vi "Avarage_measurements.vi"() -> ()   [LabVIEW 2015]
uses:
  <vilib>/Analysis/NI_AALBase.lvlib
panel:
  out "output cluster 2":T1
  out "output cluster":T1
  in  "Measurement Arrays 2":T1
  in  "Measurement Arrays":T2
  out "Stdev Measurements":T2
  out "Averaged Measurements":T2
  out "Change index":u16[](array[numeric])
  out "N":u16
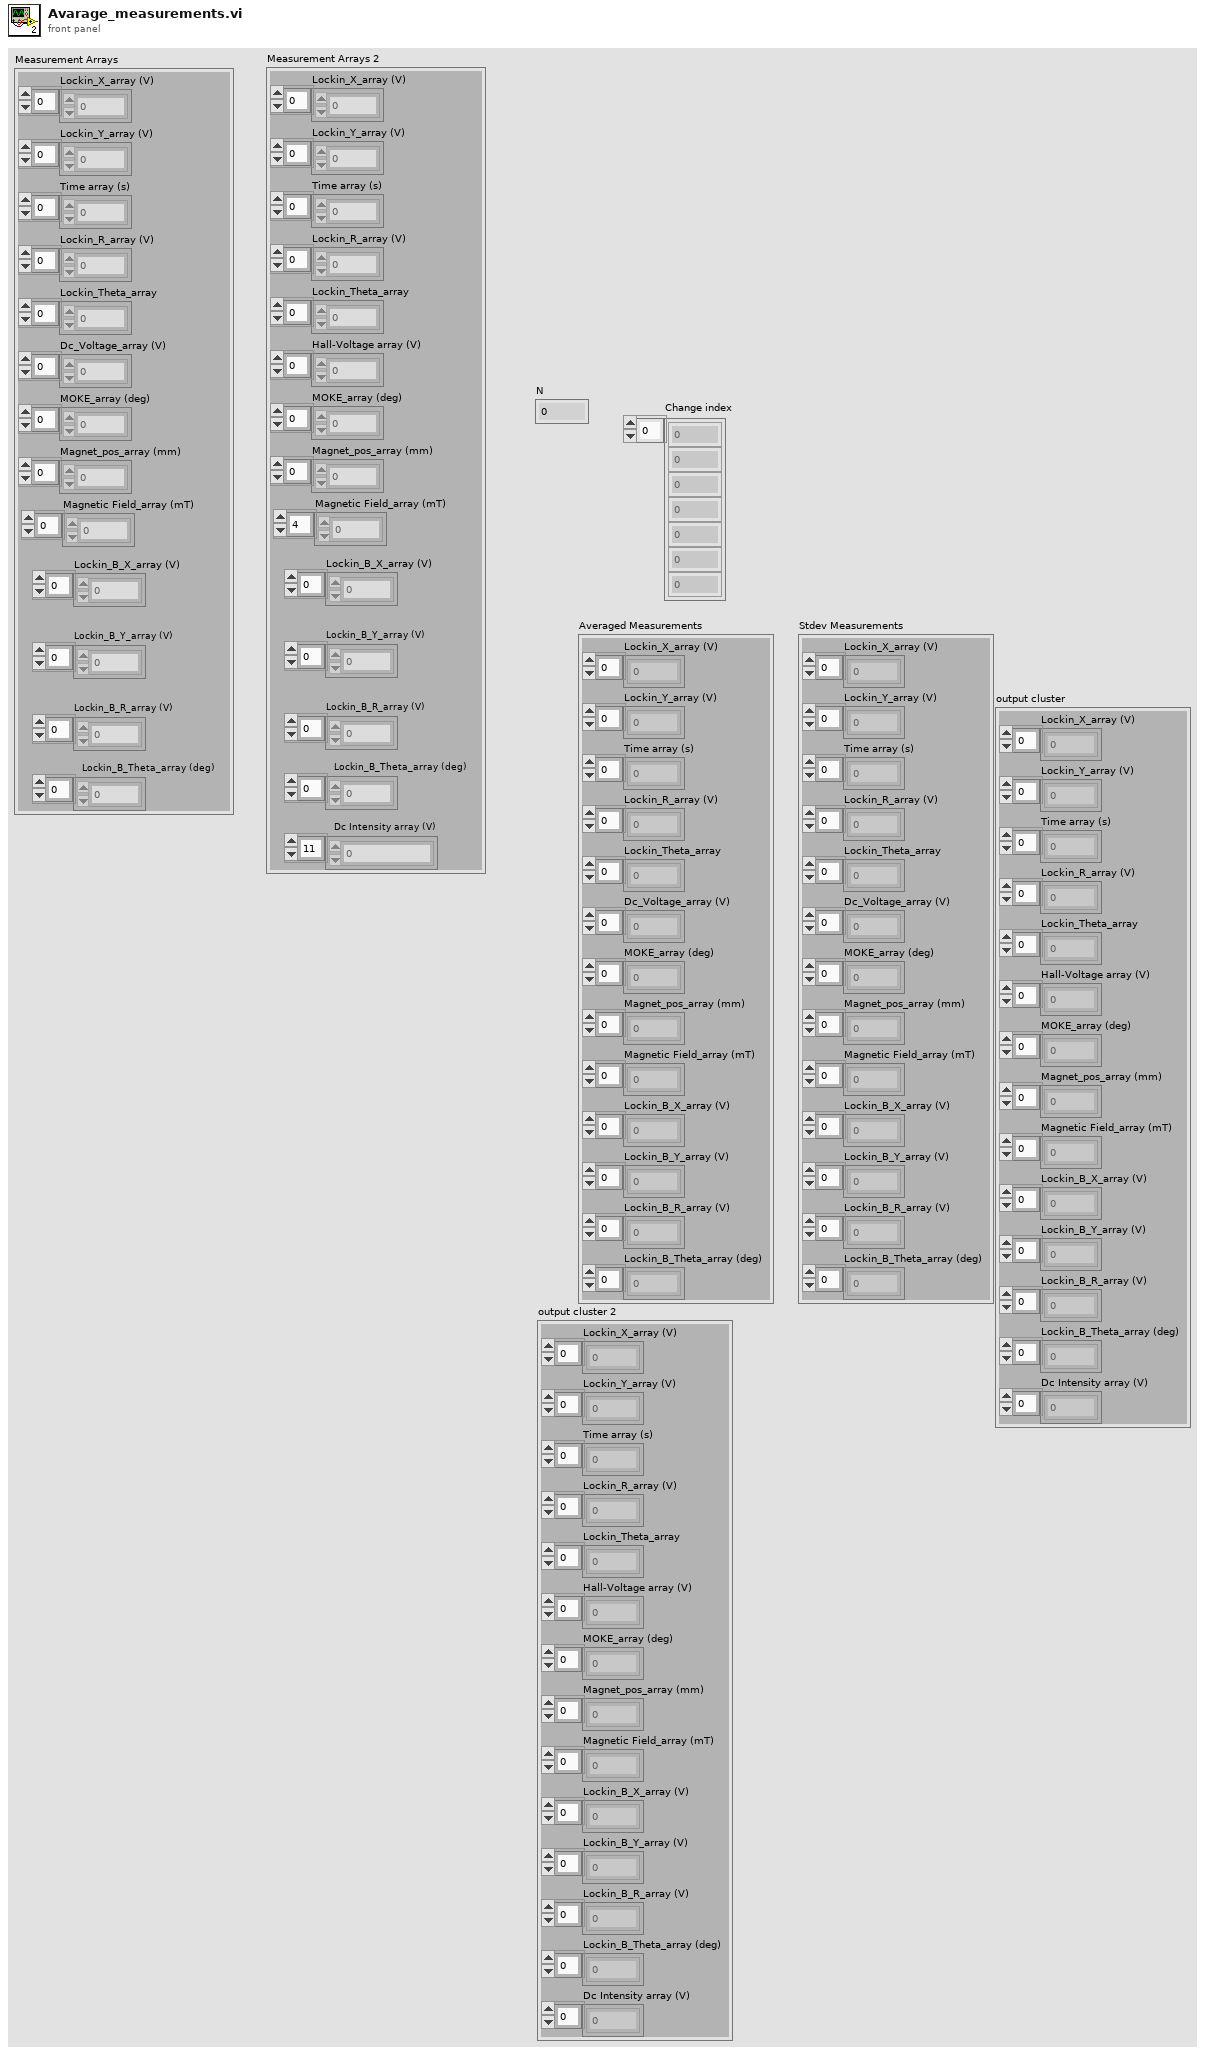
[diagram p1: front panel]
types:
  T1 = cluster{"Lockin_X_array (V)":dbl[], "Lockin_Y_array (V)":dbl[], "Time array (s)":dbl[], "Lockin_R_array (V)":dbl[], "Lockin_Theta_array":dbl[], "Hall-Voltage array (V)":dbl[], "MOKE_array (deg)":dbl[], "Magnet_pos_array (mm)":dbl[], "Magnetic Field_array (mT)":dbl[], "Lockin_B_X_array (V)":dbl[], "Lockin_B_Y_array (V)":dbl[], "Lockin_B_R_array (V)":dbl[], "Lockin_B_Theta_array (deg)":dbl[], "Dc Intensity array (V)":dbl[]}
  T2 = cluster{"Lockin_X_array (V)":dbl[], "Lockin_Y_array (V)":dbl[], "Time array (s)":dbl[], "Lockin_R_array (V)":dbl[], "Lockin_Theta_array":dbl[], "Dc_Voltage_array (V)":dbl[], "MOKE_array (deg)":dbl[], "Magnet_pos_array (mm)":dbl[], "Magnetic Field_array (mT)":dbl[], "Lockin_B_X_array (V)":dbl[], "Lockin_B_Y_array (V)":dbl[], "Lockin_B_R_array (V)":dbl[], "Lockin_B_Theta_array (deg)":dbl[]}
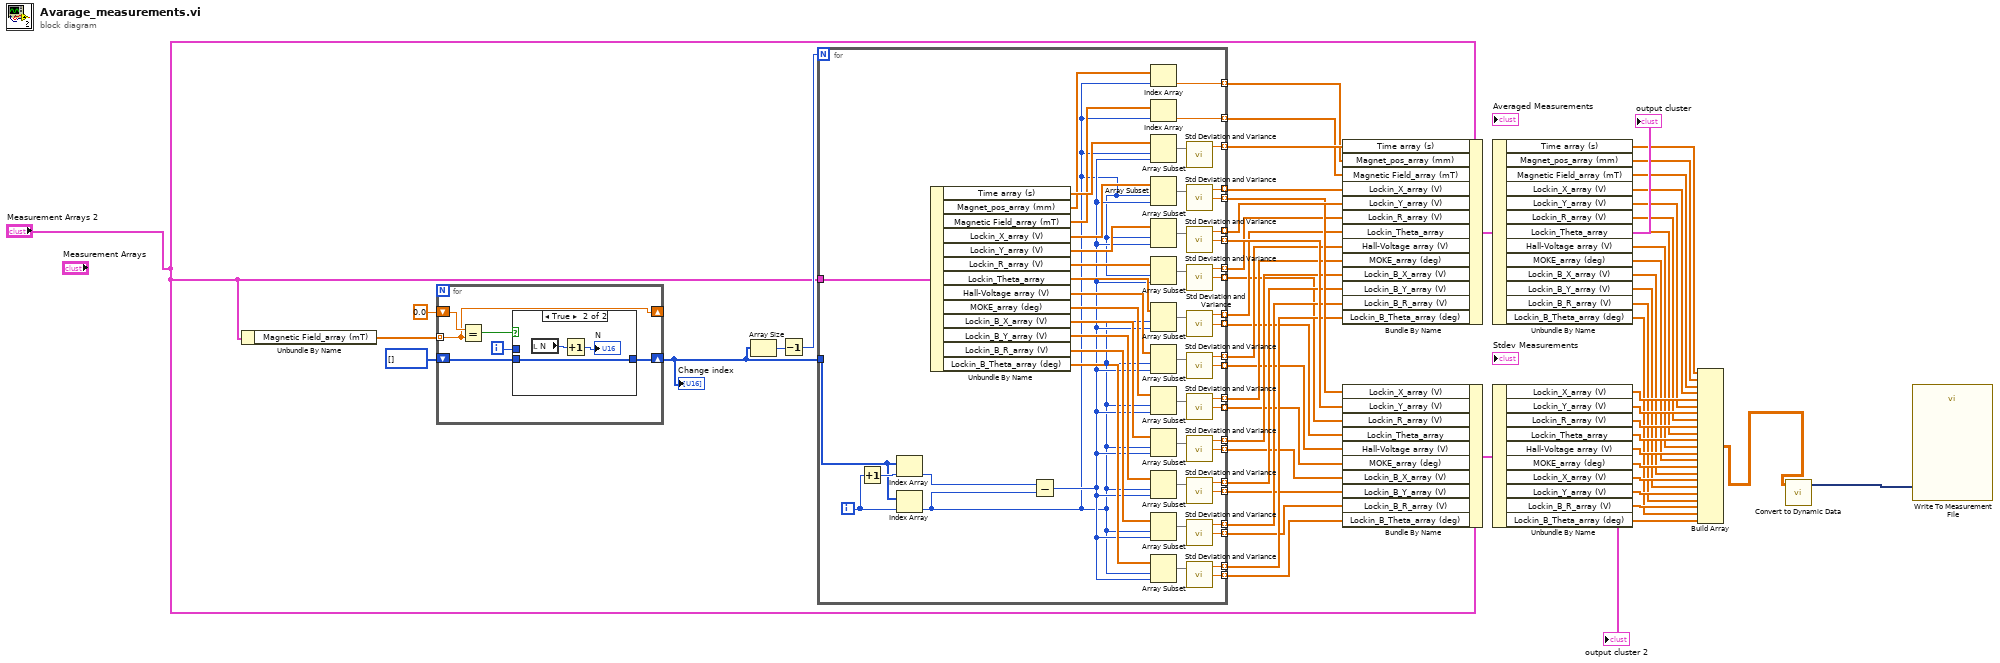
[diagram p0: block diagram]
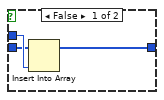
[diagram p2: hidden frame]
diagram:
  n1 = Unbundle By Name("Measurement Arrays 2") -> ("Magnetic Field_array (mT)"=w57:dbl[])
  n2 = for {
    tunnel: w57 -> [w61] mode=indexing
    shift-right: [w61] -> _
    shift-left: 0.0 ("Numeric") -> [w63]
    shift-right: [w59] -> w52
    shift-left: u16[] [] -> [w58]
    i -> [w60]
    n3 = Equal?(x=w63, y=w61) -> (x = y?=w62:bool)
    n4 = case shown="True" w62 {
      tunnel: w60 -> [w66 _]
      tunnel: [w65 w67] -> w59
      tunnel: w58 -> [w64 w67]
      frame False {
        n5 = Insert Into Array(array=w64, new element=w66) -> (w65:u16[])  [unwired: 1 in]
      }
      frame True {
        n6 = local read "N"() -> (w68:u16)
        n7 = Increment(x=w68) -> (x+1=→"N":u16)
      }
    }
  }
  "Change index" <- w52
  n8 = Array Size(array=w52) -> (size(s)=w54:i32)
  n9 = Decrement(x=w54) -> (x-1=w53:i32)
  n10 = for {
    N: w53 -> [_]
    tunnel: "Measurement Arrays 2" -> [w123]
    tunnel: w52 -> [w120]
    tunnel: [w100] -> w51 mode=indexing
    tunnel: [w99] -> w49 mode=indexing
    tunnel: [w98] -> w50 mode=indexing
    tunnel: [w97] -> w48 mode=indexing
    tunnel: [w96] -> w47 mode=indexing
    tunnel: [w95] -> w39 mode=indexing
    tunnel: [w94] -> w46 mode=indexing
    tunnel: [w93] -> w38 mode=indexing
    tunnel: [w92] -> w45 mode=indexing
    tunnel: [w91] -> w37 mode=indexing
    tunnel: [w90] -> w44 mode=indexing
    tunnel: [w89] -> w36 mode=indexing
    tunnel: [w88] -> w43 mode=indexing
    tunnel: [w87] -> w35 mode=indexing
    tunnel: [w86] -> w42 mode=indexing
    tunnel: [w85] -> w34 mode=indexing
    tunnel: [w84] -> w41 mode=indexing
    tunnel: [w83] -> w33 mode=indexing
    tunnel: [w82] -> w40 mode=indexing
    tunnel: [w81] -> w32 mode=indexing
    tunnel: [w74] -> w30 mode=indexing
    tunnel: [w73] -> w29 mode=indexing
    tunnel: [w71] -> w31 mode=indexing
    i -> [w76]
    n11 = Increment(x=w76) -> (x+1=w121:i32)
    n12 = Index Array(array=w120, index=w121) -> (element=w119:u16)
    n13 = Index Array(array=w120, index=w76) -> (element=w70:u16)
    n14 = Unbundle By Name(w123) -> ("Time array (s)"=w79:dbl[], "Magnet_pos_array (mm)"=w78:dbl[], "Magnetic Field_array (mT)"=w77:dbl[], "Lockin_X_array (V)"=w122:dbl[], "Lockin_Y_array (V)"=w118:dbl[], "Lockin_R_array (V)"=w117:dbl[], "Lockin_Theta_array"=w116:dbl[], "Hall-Voltage array (V)"=w115:dbl[], "MOKE_array (deg)"=w114:dbl[], "Lockin_B_X_array (V)"=w113:dbl[], "Lockin_B_Y_array (V)"=w112:dbl[], "Lockin_B_R_array (V)"=w111:dbl[], "Lockin_B_Theta_array (deg)"=w80:dbl[])
    n15 = Subtract(x=w119, y=w70) -> (x-y=w75:u16)
    n16 = Index Array(array=w78, index=w70) -> (element=w74:dbl)
    n17 = Index Array(array=w77, index=w70) -> (element=w73:dbl)
    n18 = Array Subset(array=w79, index=w70, length=w75) -> (w72:dbl[])
    n19 = Array Subset(array=w122, index=w70, length=w75) -> (w110:dbl[])
    n20 = Array Subset(array=w118, index=w70, length=w75) -> (w109:dbl[])
    n21 = Array Subset(array=w117, index=w70, length=w75) -> (w108:dbl[])
    n22 = Array Subset(array=w116, index=w70, length=w75) -> (w107:dbl[])
    n23 = Array Subset(array=w115, index=w70, length=w75) -> (w106:dbl[])
    n24 = Array Subset(array=w114, index=w70, length=w75) -> (w105:dbl[])
    n25 = Array Subset(array=w113, index=w70, length=w75) -> (w104:dbl[])
    n26 = Array Subset(array=w112, index=w70, length=w75) -> (w103:dbl[])
    n27 = Array Subset(array=w111, index=w70, length=w75) -> (w102:dbl[])
    n28 = Array Subset(array=w80, index=w70, length=w75) -> (w101:dbl[])
    n29 = call <vilib>:"Std Deviation and Variance.vi"("X"=w72) -> ("mean"=w71:dbl)  [unwired: 1 in, 2 out]
    n30 = call <vilib>:"Std Deviation and Variance.vi"("X"=w110) -> ("mean"=w100:dbl, "standard deviation"=w99:dbl)  [unwired: 1 in, 1 out]
    n31 = call <vilib>:"Std Deviation and Variance.vi"("X"=w109) -> ("mean"=w98:dbl, "standard deviation"=w97:dbl)  [unwired: 1 in, 1 out]
    n32 = call <vilib>:"Std Deviation and Variance.vi"("X"=w108) -> ("mean"=w96:dbl, "standard deviation"=w95:dbl)  [unwired: 1 in, 1 out]
    n33 = call <vilib>:"Std Deviation and Variance.vi"("X"=w107) -> ("mean"=w94:dbl, "standard deviation"=w93:dbl)  [unwired: 1 in, 1 out]
    n34 = call <vilib>:"Std Deviation and Variance.vi"("X"=w106) -> ("mean"=w92:dbl, "standard deviation"=w91:dbl)  [unwired: 1 in, 1 out]
    n35 = call <vilib>:"Std Deviation and Variance.vi"("X"=w105) -> ("mean"=w90:dbl, "standard deviation"=w89:dbl)  [unwired: 1 in, 1 out]
    n36 = call <vilib>:"Std Deviation and Variance.vi"("X"=w104) -> ("mean"=w88:dbl, "standard deviation"=w87:dbl)  [unwired: 1 in, 1 out]
    n37 = call <vilib>:"Std Deviation and Variance.vi"("X"=w103) -> ("mean"=w86:dbl, "standard deviation"=w85:dbl)  [unwired: 1 in, 1 out]
    n38 = call <vilib>:"Std Deviation and Variance.vi"("X"=w102) -> ("mean"=w84:dbl, "standard deviation"=w83:dbl)  [unwired: 1 in, 1 out]
    n39 = call <vilib>:"Std Deviation and Variance.vi"("X"=w101) -> ("mean"=w82:dbl, "standard deviation"=w81:dbl)  [unwired: 1 in, 1 out]
  }
  n40 = Bundle By Name(cluster="Measurement Arrays 2", "Time array (s)"=w31, "Magnet_pos_array (mm)"=w30, "Magnetic Field_array (mT)"=w29, "Lockin_X_array (V)"=w51, "Lockin_Y_array (V)"=w50, "Lockin_R_array (V)"=w47, "Lockin_Theta_array"=w46, "Hall-Voltage array (V)"=w45, "MOKE_array (deg)"=w44, "Lockin_B_X_array (V)"=w43, "Lockin_B_Y_array (V)"=w42, "Lockin_B_R_array (V)"=w41, "Lockin_B_Theta_array (deg)"=w40) -> (w28:T1)
  "output cluster" <- w28
  n41 = Bundle By Name(cluster="Measurement Arrays 2", "Lockin_X_array (V)"=w49, "Lockin_Y_array (V)"=w48, "Lockin_R_array (V)"=w39, "Lockin_Theta_array"=w38, "Hall-Voltage array (V)"=w37, "MOKE_array (deg)"=w36, "Lockin_B_X_array (V)"=w35, "Lockin_B_Y_array (V)"=w34, "Lockin_B_R_array (V)"=w33, "Lockin_B_Theta_array (deg)"=w32) -> (w27:T1)
  "output cluster 2" <- w27
  n42 = Unbundle By Name(w28) -> ("Time array (s)"=w26:dbl[], "Magnet_pos_array (mm)"=w25:dbl[], "Magnetic Field_array (mT)"=w24:dbl[], "Lockin_X_array (V)"=w22:dbl[], "Lockin_Y_array (V)"=w20:dbl[], "Lockin_R_array (V)"=w19:dbl[], "Lockin_Theta_array"=w17:dbl[], "Hall-Voltage array (V)"=w15:dbl[], "MOKE_array (deg)"=w13:dbl[], "Lockin_B_X_array (V)"=w11:dbl[], "Lockin_B_Y_array (V)"=w9:dbl[], "Lockin_B_R_array (V)"=w7:dbl[], "Lockin_B_Theta_array (deg)"=w5:dbl[])
  n43 = Unbundle By Name(w27) -> ("Lockin_X_array (V)"=w23:dbl[], "Lockin_Y_array (V)"=w21:dbl[], "Lockin_R_array (V)"=w18:dbl[], "Lockin_Theta_array"=w16:dbl[], "Hall-Voltage array (V)"=w14:dbl[], "MOKE_array (deg)"=w12:dbl[], "Lockin_X_array (V)"=w10:dbl[], "Lockin_Y_array (V)"=w8:dbl[], "Lockin_B_R_array (V)"=w6:dbl[], "Lockin_B_Theta_array (deg)"=w4:dbl[])
  n44 = Build Array(w26, w25, w24, w22, w23, w20, w21, w19, w18, w17, w16, w15, w14, w13, w12, w11, w10, w9, w8, w7, w6, w5, w4) -> (w2:dbl[][])
  n45 = call "Convert to Dynamic Data"("2D Array"=w2) -> ("Dynamic Data Type"=w3:dynamicdata)  [unwired: 3 in]
  n46 = call "Write To Measurement File"("Signals"=w3) -> ()  [unwired: 16 in, 3 out]
